vi "CollideWithBorder.vi"(7 "UpDownLeftRightBounce":dbl[](array[numeric])=[1.0, 1.0, 1.0, 1.0], 8 "error in (no error)":errorcluster, 10 "UpDownLeftRightCollide":bool[](array[boolean]), 11 "Object in":refnum<class "GameObject.lvclass">) -> (0 "error out":errorcluster, 2 "collided?":bool, 3 "Object out":refnum<class "GameObject.lvclass">)   [LabVIEW 2019, in "RT_Game.lvlib" / "GameObject.lvclass"]
uses:
  GameObject/GameObject.lvclass
  Velocity.ctl
  GameObject/GameObject.lvclass/GameObject.ctl
  Globals.vi
  RT_Game.lvlib
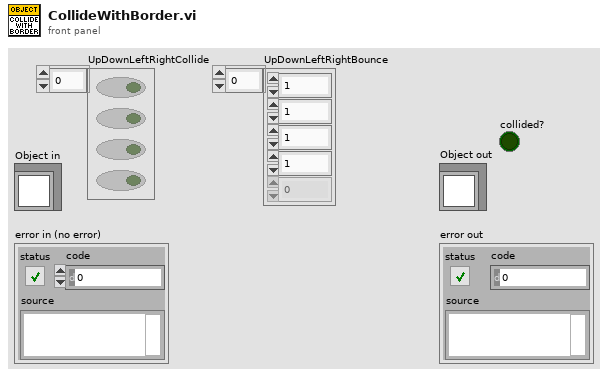
[diagram p1: front panel]
types:
  T1 = typedef "RT_Game.lvlib/Velocity.ctl" = cluster{"x":dbl, "y":dbl}
  T2 = typedef "RT_Game.lvlib/Game.lvclass/Coordinate.ctl" = cluster{"x":dbl, "y":dbl}
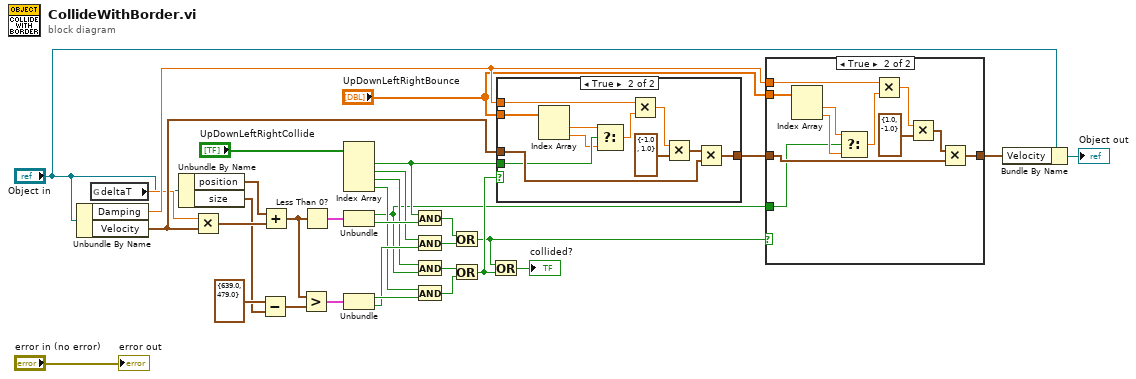
[diagram p0: block diagram]
diagram:
  n1 = Unbundle By Name("Object in") -> ("Damping"=w33:dbl, "Velocity"=w31:T1)
  n2 = global read "Globals.vi" "deltaT"() -> (w27:dbl)
  n3 = Unbundle By Name("Object in") -> ("position"=w15:T2, "size"=w14:T2)
  n4 = Multiply(x=w27, y=w31) -> (x*y=w26:T1)
  n5 = Subtract(x=T1 {"x"=639.0, "y"=479.0} ("y"), y=w14) -> (x-y=w28:T1)
  n6 = Add(x=w15, y=w26) -> (x+y=w20:T2)
  n7 = Greater?(x=w20, y=w28) -> (0:w22:cluster{"x":bool, "y":bool})
  n8 = Less Than 0?(x=w20) -> (x < 0?=w19:cluster{"x":bool, "y":bool})
  n9 = Index Array(array="UpDownLeftRightCollide") -> (element #1=w3:bool, element #2=w6:bool, element #3=w5:bool, element #4=w4:bool)  [unwired: 4 in]
  n10 = Unbundle(w19) -> ("x"=w1:bool, "y"=w23:bool)
  n11 = Unbundle(w22) -> ("x"=w29:bool, "y"=w24:bool)
  n12 = And(x=w3, y=w23) -> (x .and. y?=w9:bool)
  n13 = And(x=w6, y=w24) -> (x .and. y?=w7:bool)
  n14 = And(x=w5, y=w1) -> (x .and. y?=w10:bool)
  n15 = And(x=w4, y=w29) -> (x .and. y?=w8:bool)
  n16 = Or(x=w9, y=w7) -> (x .or. y?=w13:bool)
  n17 = Or(x=w10, y=w8) -> (x .or. y?=w30:bool)
  n18 = Or(x=w13, y=w30) -> (x .or. y?=→"collided?":bool)
  n19 = case shown="True" w30 {
    tunnel: w31 -> [w34 w45]
    tunnel: [w34 w43] -> w32
    tunnel: w33 -> [_ w41]
    tunnel: w3 -> [_ w40]
    tunnel: "UpDownLeftRightBounce" -> [_ w39]
    frame False {
    }
    frame True {
      n20 = Index Array(array=w39) -> (element #1=w38:dbl, element #2=w37:dbl)  [unwired: 2 in]
      n21 = Select(t=w38, s=w40, f=w37) -> (s? t:f=w35:dbl)
      n22 = Multiply(x=w41, y=w35) -> (x*y=w36:dbl)
      n23 = Multiply(x=w36, y=T1 {"x"=-1.0, "y"=1.0} ("x")) -> (x*y=w42:T1)
      n24 = Multiply(x=w42, y=w45) -> (x*y=w43:T1)
    }
  }
  n25 = case shown="True" w13 {
    tunnel: w32 -> [w46 w57]
    tunnel: [w46 w55] -> w17
    tunnel: w33 -> [_ w53]
    tunnel: "UpDownLeftRightBounce" -> [_ w50]
    tunnel: w1 -> [_ w49]
    frame False {
    }
    frame True {
      n26 = Index Array(array=w50) -> (element #1=w51:dbl, element #2=w52:dbl)  [unwired: 2 in]
      n27 = Select(t=w51, s=w49, f=w52) -> (s? t:f=w47:dbl)
      n28 = Multiply(x=w53, y=w47) -> (x*y=w48:dbl)
      n29 = Multiply(x=w48, y=T1 {"x"=1.0, "y"=-1.0} ("x")) -> (x*y=w54:T1)
      n30 = Multiply(x=w54, y=w57) -> (x*y=w55:T1)
    }
  }
  n31 = Bundle By Name(cluster="Object in", "Velocity"=w17) -> (→"Object out":refnum<class "GameObject.lvclass">)
  "error out" <- "error in (no error)"
